vi "Robot Global Data.vi"() -> ()   [LabVIEW 2017]
doc: "This global VI can contain as many global variables as you need. Place a control on the panel, give it a good name. To read or write to it from a VI, drag the icon to the diagram of that VI. You can also drag from the project. Click on the node to change which global you access. You shouldn't have multiple locations writing to a global or it will cause a race-condition."
uses:
  <vilib>/Rock Robotics/WPI/Camera/WPI_CameraImageSize.ctl
  <vilib>/Rock Robotics/WPI/DriverStation/WPI_DriverStationRobotMode2.ctl
panel:
  in  "Reset Wheels":bool
  in  "Has Cube":bool
  in  "Reset Arm":bool
  in  "Reset Gyro":bool
  in  "Autonomous Outputs":cluster{"X":dbl, "Y":dbl, "Z":dbl}
  in  "Desired Elbow":dbl
  in  "Desired Shoulder":dbl
  in  "Current Parametric Position":dbl
  in  "Desired Parametric Position":dbl
  in  "Current Elbow":dbl
  in  "Current Shoulder":dbl
  in  "Next Destination Position":i32
  in  "Current Destination Position":i32
  in  "Current State":i32
  in  "Torque Weighting":T1={"Forearm importance"=0.001338096, "Backarm importance"=0.000314995}
  in  "Robot Geometry":T2={"Forearm Length"=23.5, "Backarm Length"=29.075, "Forearm Center of Gravity Length"=9.25, "Backarm Center of Gravity Length"=10.625, "Weight of Cube"=3.2, "Weight of Forearm"=5.3, "Weight of Backarm"=9.4}
  in  "Solenoid 4/Extra":bool
  in  "Solenoid 3/Grabber":bool
  in  "Solenoid 2/Elbow":bool
  in  "Solenoid 1/Shoulder":bool
  in  "Arm Powers":dbl[](array[numeric])
  in  "Controller":T3
  in  "Robot Mode":T4
  in  "image size":T5=enum."320x240"
  in  "Enable Vision":bool
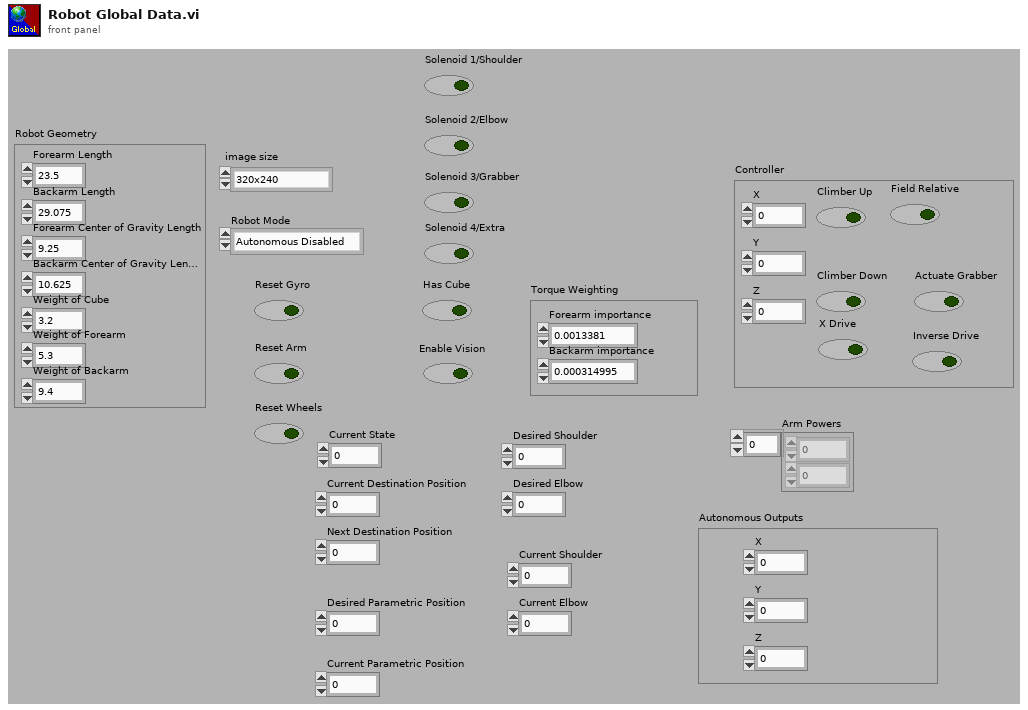
[diagram p1: front panel]
types:
  T1 = cluster{"Forearm importance":dbl, "Backarm importance":dbl}
  T2 = cluster{"Forearm Length":dbl, "Backarm Length":dbl, "Forearm Center of Gravity Length":dbl, "Backarm Center of Gravity Length":dbl, "Weight of Cube":dbl, "Weight of Forearm":dbl, "Weight of Backarm":dbl}
  T3 = cluster{"X":dbl, "Y":dbl, "Z":dbl, "Climber Down":bool, "Climber Up":bool, "X Drive":bool, "Field Relative":bool, "Actuate Grabber":bool, "Inverse Drive":bool}
  T4 = typedef "WPI_DriverStationRobotMode2.ctl" = enum16{"Autonomous Disabled", "Autonomous Enabled", "Teleop Disabled", "Teleop Enabled", "Disconnected", "Finish", "Test Disabled", "Test Enabled", "Emergency Stopped"}
  T5 = typedef "WPI_CameraImageSize.ctl" = enum16{"640x480", "320x240", "160x120", "Custom"}
diagram:
